vi "CreateGUID(冲突时的文件备份2013-03-27 14-08-05).vi"(8 "错误输入":errorcluster) -> (0 "错误输出":errorcluster, 3 "Create GUID":string)   [LabVIEW 2012, in "Application.lvlib"]
uses:
  Application.lvlib
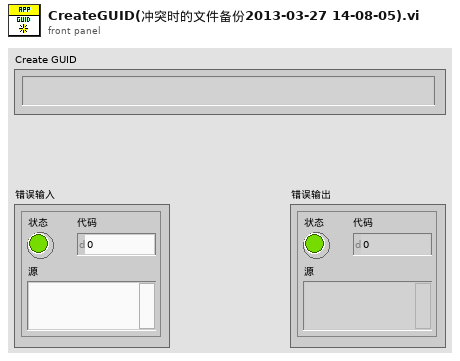
[diagram p1: front panel]
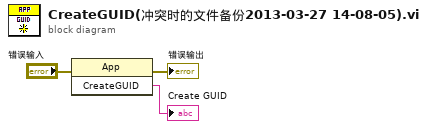
[diagram p0: block diagram]
diagram:
  n1 = invoke class="App" method="CreateGUID"(error in="错误输入") -> (error out=→"错误输出":errorcluster, "CreateGUID"=→"Create GUID":string)  [unwired: 2 in, 1 out]
